vi "Main - Round Decimal Places.vi"(7 "DecimalPlaces":u8, 11 "Number to round":dbl=1234.56789 format="%_9f") -> (3 "Rounded number":dbl=1235.0 format="%_9f")   [LabVIEW 2019]
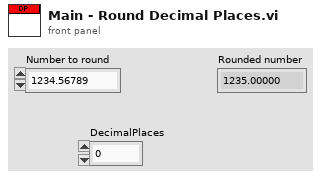
[diagram p1: front panel]
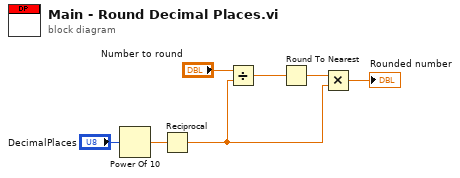
[diagram p0: block diagram]
diagram:
  n1 = Power Of 10(x="DecimalPlaces") -> (10^x=w3:dbl)
  n2 = Reciprocal(x=w3) -> (1/x=w2:dbl)
  n3 = Divide(x="Number to round", y=w2) -> (x/y=w6:dbl)
  n4 = Round To Nearest(number=w6) -> (nearest integer value=w5:dbl)
  n5 = Multiply(x=w5, y=w2) -> (x*y=→"Rounded number":dbl)
